vi "MainTemplate.vi"() -> ()   [LabVIEW 2019]
uses:
  Application_class/Application.lvclass
  <vilib>/Utility/error.llb/Error Cluster From Error Code.vi
  <vilib>/ErrorRing/Error Ring.xnode
panel:
  out "Display <Replace Me> 2":string
  out "Display <Replace Me>":string
  in  "Exit":bool
  in  "Inject Error<Replace Me>":bool
  in  "Do Something <Replace Me>":bool
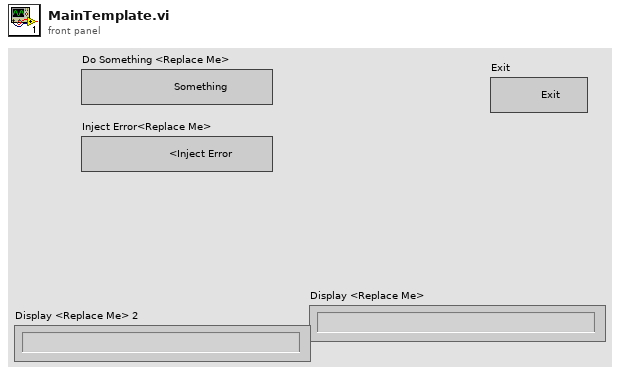
[diagram p1: front panel]
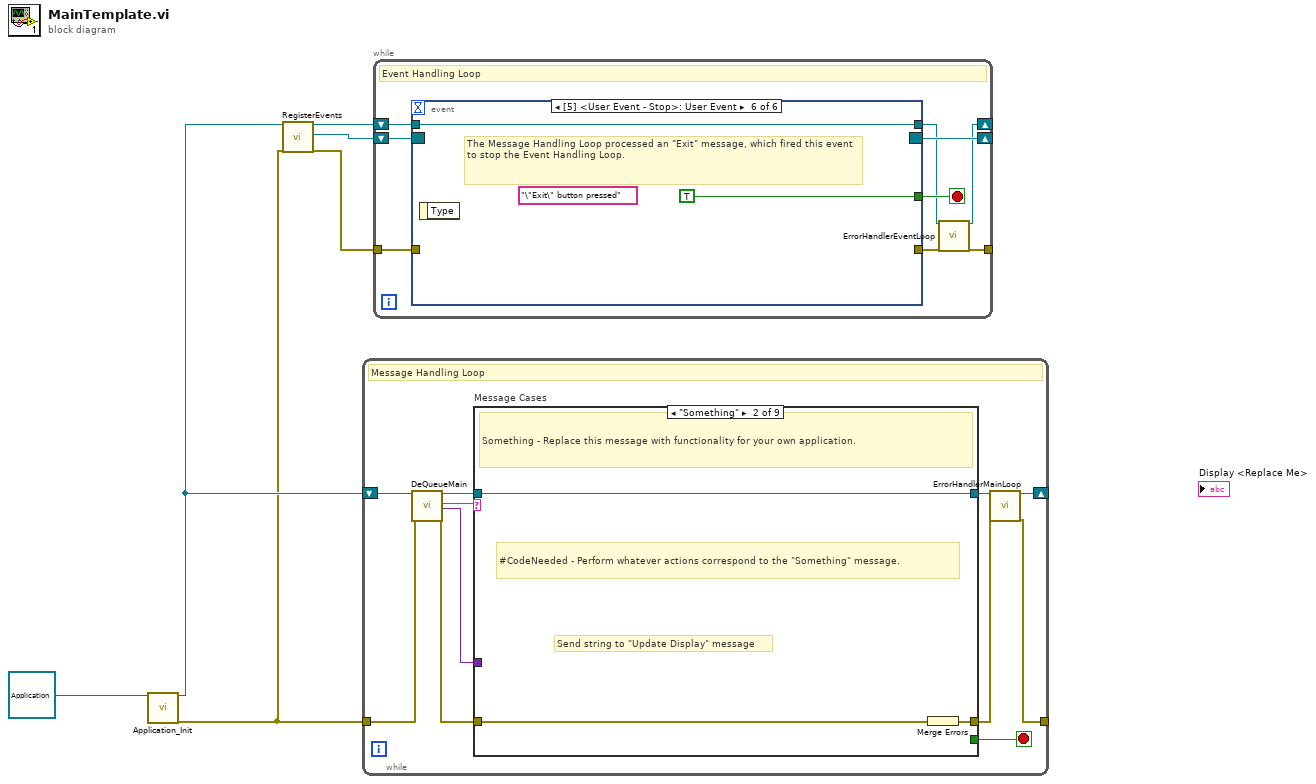
[diagram p0: block diagram]
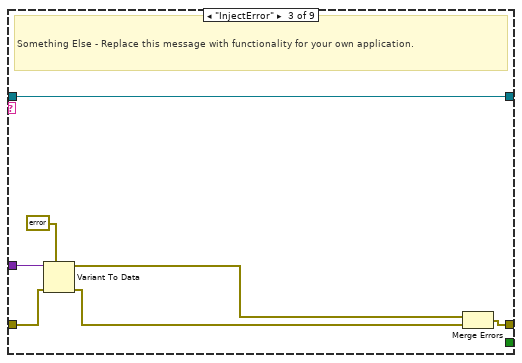
[diagram p3: hidden frame]
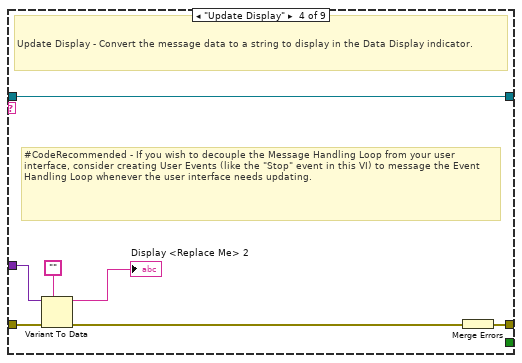
[diagram p4: hidden frame]
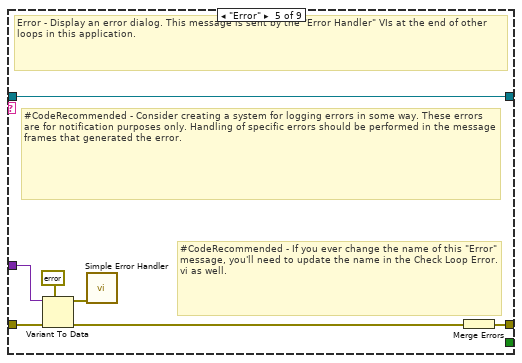
[diagram p5: hidden frame]
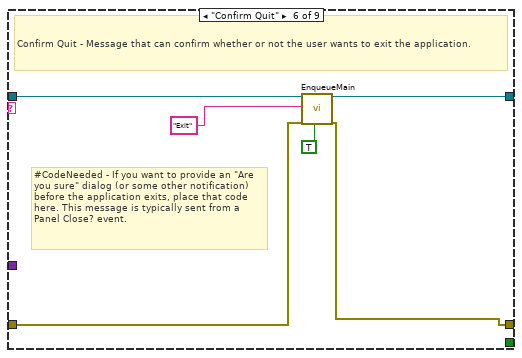
[diagram p6: hidden frame]
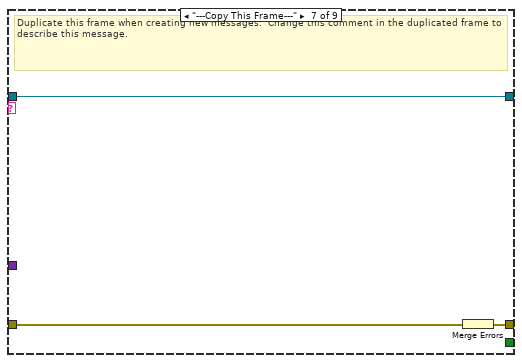
[diagram p7: hidden frame]
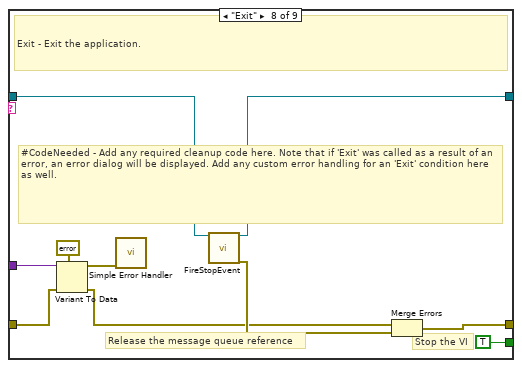
[diagram p8: hidden frame]
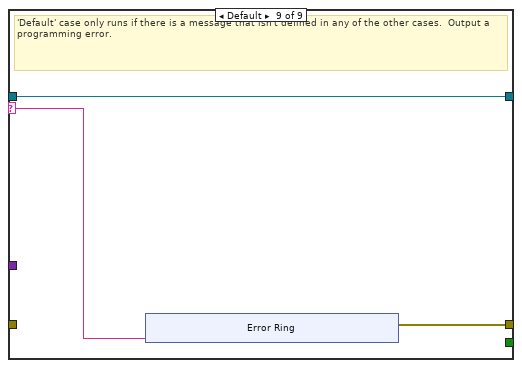
[diagram p9: hidden frame]
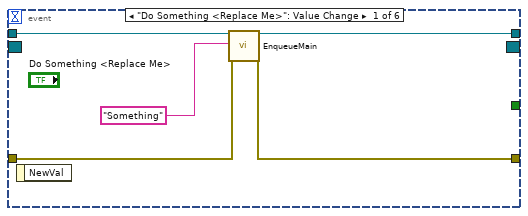
[diagram p10: hidden frame]
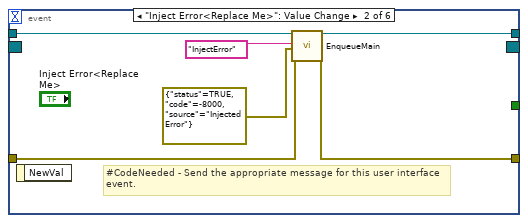
[diagram p11: hidden frame]
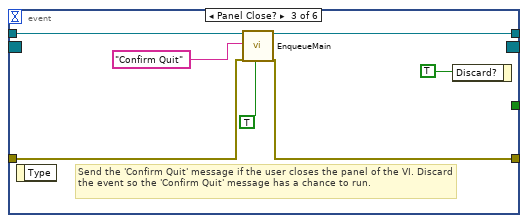
[diagram p12: hidden frame]
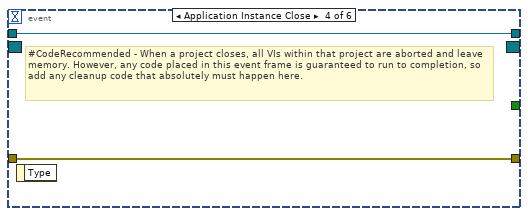
[diagram p13: hidden frame]
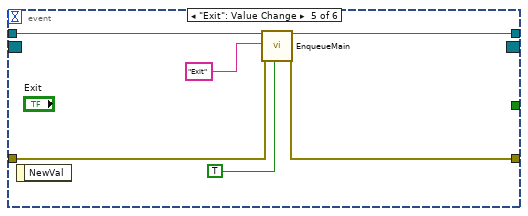
[diagram p14: hidden frame]
diagram:
  n1 = call "Application_Init.vi"("object in"=refnum<class "Application.lvclass"> refnum ("Application")) -> ("object out"=w2:refnum<class "Application.lvclass">, "error out"=w1:errorcluster)  [unwired: 17 in]
  n2 = call-dynamic "RegisterEvents.vi"("object in"=w2, "error in (no error)"=w1) -> ("object out"=w4:refnum<class "Application.lvclass">, "Event Registration Refnum"=w5:refnum<event-registration>, "error out"=w3:errorcluster)  [unwired: 15 in]
  n3 = while {
    tunnel: w1 -> [w7]
    tunnel: [w11] -> _
    shift-right: [w10] -> _
    shift-left: w2 -> [w16]
    stop <- w17 stop-if-true
    # "Message Handling Loop"
    n4 = call-dynamic "DeQueueMain.vi"("object in"=w16, "error in (no error)"=w7) -> ("object out"=w15:refnum<class "Application.lvclass">, "Message"=w14:string, "Message Data"=w13:variant, "error out"=w8:errorcluster)  [unwired: 14 in]
    n5 = case "Message Cases" shown="\"Something\"" w14 {
      selector: w14 -> [_ _ _ _ _ _ _ _ w64]
      tunnel: w8 -> [w19 w21 w24 w35 w43 w49 w52 w53 _]
      tunnel: [w19 w22 w29 w36 w38 w48 w51 w61 w65] -> w12
      tunnel: [_ _ _ _ _ _ _ TRUE _] -> w17
      tunnel: w13 -> [_ _ w27 w34 w42 _ _ w58 _]
      tunnel: w15 -> [w18 w20 w28 w30 w37 w45 w50 w56 w63]
      tunnel: [w18 w20 w28 w30 w37 w46 w50 w57 w63] -> w9
      frame "Initialize" {
        # "Initialize - All initialization work should take place in this message, since other loops can potentially enqueue messages that execute immediately after this one."
      }
      frame "Something" {
        # "Send string to \"Update Display\" message"
        # "#CodeNeeded - Perform whatever actions correspond to the \"Something\" message."
        # "Something - Replace this message with functionality for your own application."
        n6 = Merge Errors(w21) -> (w22:errorcluster)
      }
      frame "InjectError" {
        # "Something Else - Replace this message with functionality for your own application."
        n7 = Variant To Data(error in=w24, type=errorcluster {"status"=FALSE, "code"=0, "source"=""} ("error in (no error)"), Variant=w27) -> (data=w23:errorcluster, error out=w25:errorcluster)
        n8 = Merge Errors(w23, w25) -> (w29:errorcluster)
      }
      frame "Update Display" {
        # "#CodeRecommended - If you wish to decouple the Message Handling Loop from your user interface, consider creating User Events (like the \"Stop\" event in this VI) to message the Event Handling Loop whenever the user interface needs updating."
        # "Update Display - Convert the message data to a string to display in the Data Display indicator."
        n9 = Variant To Data(error in=w35, type="", Variant=w34) -> (data=→"Display <Replace Me> 2":string, error out=w32:errorcluster)
        n10 = Merge Errors(w32) -> (w36:errorcluster)
      }
      frame "Error" {
        # "#CodeRecommended - If you ever change the name of this \"Error\" message, you'll need to update the name in the Check Loop Error.vi as well."
        # "#CodeRecommended - Consider creating a system for logging errors in some way. These errors are for notification purposes only. Handling of specific errors should be performed in the message frames that generated the error."
        # "Error - Display an error dialog. This message is sent by the \"Error Handler\" VIs at the end of other loops in this application."
        n11 = Variant To Data(error in=w43, type=errorcluster {"status"=FALSE, "code"=0, "source"=""} ("error constant"), Variant=w42) -> (data=w40:errorcluster, error out=w39:errorcluster)
        n12 = call <vilib>:"Simple Error Handler.vi"("error in (no error)"=w40) -> ()  [unwired: 4 in, 5 out]
        n13 = Merge Errors(w39) -> (w38:errorcluster)
      }
      frame "Confirm Quit" {
        # "#CodeNeeded - If you want to provide an \"Are you sure\" dialog (or some other notification) before the application exits, place that code here. This message is typically sent from a Panel Close? event."
        # "Confirm Quit - Message that can confirm whether or not the user wants to exit the application."
        n14 = call-dynamic "EnqueueMain.vi"("object in"=w45, "Message"="Exit", "error in (no error)"=w49, "Priority Message? (F)"=TRUE) -> ("object out"=w46:refnum<class "Application.lvclass">, "error out"=w48:errorcluster)  [unwired: 14 in]
      }
      frame "---Copy This Frame---" {
        # "Duplicate this frame when creating new messages.  Change this comment in the duplicated frame to describe this message."
        n15 = Merge Errors(w52) -> (w51:errorcluster)
      }
      frame "Exit" {
        # "Stop the VI"
        # "Release the message queue reference"
        # "#CodeNeeded - Add any required cleanup code here. Note that if 'Exit' was called as a result of an error, an error dialog will be displayed. Add any custom error handling for an 'Exit' condition here as well."
        # "Exit - Exit the application."
        n16 = Variant To Data(error in=w53, type=errorcluster {"status"=FALSE, "code"=0, "source"=""} ("error constant"), Variant=w58) -> (data=w59:errorcluster, error out=w54:errorcluster)
        n17 = call <vilib>:"Simple Error Handler.vi"("error in (no error)"=w59) -> ()  [unwired: 4 in, 5 out]
        n18 = call-dynamic "FireStopEvent.vi"("object in"=w56) -> ("object out"=w57:refnum<class "Application.lvclass">, "error out"=w55:errorcluster)  [unwired: 17 in]
        n19 = Merge Errors(w54, w55) -> (w61:errorcluster)
      }
      frame Default {
        # "'Default' case only runs if there is a message that isn't defined in any of the other cases.  Output a programming error."
        n20 = xnode "Error Ring"("parameter 0"=w64) -> ("error out"=w65:errorcluster)
      }
    }
    n21 = call-dynamic "ErrorHandlerMainLoop.vi"("object in"=w9, "error in (no error)"=w12) -> ("object out"=w10:refnum<class "Application.lvclass">, "error out"=w11:errorcluster)  [unwired: 16 in]
  }
  n22 = while {
    shift-right: [w80] -> _
    shift-left: w5 -> [w81]
    tunnel: [w75] -> _
    shift-right: [w73] -> _
    shift-left: w4 -> [w78]
    tunnel: w3 -> [w77]
    stop <- w79 stop-if-true
    # "Event Handling Loop"
    n23 = event shown="[5] <User Event - Stop>: User Event" {
      selector: w81 -> [_ _ _ _ _ _]
      dyn-events: [_ _ _ _ _ _] -> w80
      timeout: _ -> [_ _ _ _ _ _]
      tunnel: [_ _ _ _ _ TRUE ("Discard?")] -> w79
      tunnel: [w83 w89 w95 w100 w102 _] -> w76
      tunnel: w78 -> [w86 w92 w94 w101 w107 w108]
      tunnel: [w85 w91 w93 w101 w106 w108] -> w74
      tunnel: w77 -> [w82 w88 w96 w100 w103 _]
      event "Do Something <Replace Me>": Value Change {
        n24 = event-data() -> ()  [unwired: 1 in, 1 out]
        n25 = call-dynamic "EnqueueMain.vi"("object in"=w86, "Message"="Something", "error in (no error)"=w82) -> ("object out"=w85:refnum<class "Application.lvclass">, "error out"=w83:errorcluster)  [unwired: 15 in]
      }
      event "Inject Error<Replace Me>": Value Change {
        # "#CodeNeeded - Send the appropriate message for this user interface event."
        n26 = event-data() -> ()  [unwired: 1 in, 1 out]
        n27 = call-dynamic "EnqueueMain.vi"("object in"=w92, "Message"="InjectError", "Message Data"=errorcluster {"status"=TRUE, "code"=-8000, "source"="Injected Error"} ("error in (no error)"), "error in (no error)"=w88) -> ("object out"=w91:refnum<class "Application.lvclass">, "error out"=w89:errorcluster)  [unwired: 14 in]
      }
      event Panel Close? {
        # "Send the 'Confirm Quit' message if the user closes the panel of the VI. Discard the event so the 'Confirm Quit' message has a chance to run."
        n28 = event-data() -> ()  [unwired: 1 in, 1 out]
        n29 = call-dynamic "EnqueueMain.vi"("object in"=w94, "Message"="Confirm Quit", "error in (no error)"=w96, "Priority Message? (F)"=TRUE) -> ("object out"=w93:refnum<class "Application.lvclass">, "error out"=w95:errorcluster)  [unwired: 14 in]
        n30 = event-data("Discard?"=TRUE) -> ()  [unwired: 1 in, 1 out]
      }
      event Application Instance Close {
        # "#CodeRecommended - When a project closes, all VIs within that project are aborted and leave memory. However, any code placed in this event frame is guaranteed to run to completion, so add any cleanup code that absolutely must happen here."
        n31 = event-data() -> ()  [unwired: 1 in, 1 out]
      }
      event "Exit": Value Change {
        n32 = event-data() -> ()  [unwired: 1 in, 1 out]
        n33 = call-dynamic "EnqueueMain.vi"("object in"=w107, "Message"="Exit", "error in (no error)"=w103, "Priority Message? (F)"=TRUE) -> ("object out"=w106:refnum<class "Application.lvclass">, "error out"=w102:errorcluster)  [unwired: 14 in]
      }
      event User Event {
        (unwired) "\"Exit\" button pressed" ("VI Stopped")
        # "The Message Handling Loop processed an \"Exit\" message, which fired this event to stop the Event Handling Loop."
        n34 = event-data() -> ()  [unwired: 1 in, 1 out]
      }
    }
    n35 = call-dynamic "ErrorHandlerEventLoop.vi"("object in"=w74, "error in (no error)"=w76) -> ("object out"=w73:refnum<class "Application.lvclass">, "error out"=w75:errorcluster)  [unwired: 16 in]
  }
